vi "Connector.vi"(8 "ErrorArray":errorcluster[](array[cluster]), 9 "remote_port":u16=60100, 10 "remote_address":string="127.0.0.1") -> (0 "ErrorArray":errorcluster[](array[cluster]))   [LabVIEW 2014, in "Comms.lvlib"]
uses:
  Comms.lvlib
  <userlib>/NIST/Socket Class/Classes/Socket.TCP/Socket.TCP.lvclass
  <userlib>/NIST/NISTErrorLib/NISTErrorLib.lvlib
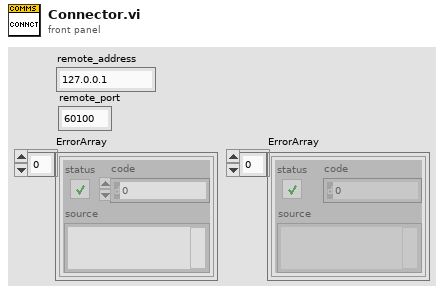
[diagram p1: front panel]
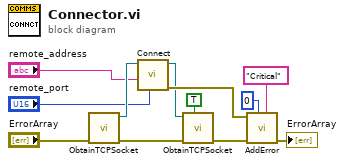
[diagram p0: block diagram]
diagram:
  n1 = call "ObtainTCPSocket.vi"("ErrorArray"="ErrorArray") -> ("ErrorArray"=w10:errorcluster[], "SocketRef"=w9:refnum<class "Socket.TCP.lvclass">)  [unwired: 9 in]
  n2 = call-dynamic "Connect.vi"("remote_port"="remote_port", "remote_address"="remote_address", "Socket.TCP in"=w9) -> ("error out"=w6:errorcluster, "Socket.TCP out"=w3:refnum<class "Socket.TCP.lvclass">)  [unwired: 7 in]
  n3 = call "ObtainTCPSocket.vi"("write (f)"=TRUE, "ErrorArray"=w10, "SocketRef"=w3) -> ("ErrorArray"=w5:errorcluster[])  [unwired: 7 in, 1 out]
  n4 = call <userlib>:"AddError.vi"("Severity"="Critical", "Priority"=u8 0, "ErrorArray"=w5, "error in (no error)"=w6) -> ("ErrorArray"=→"ErrorArray":errorcluster[])  [unwired: 6 in, 1 out]
